vi "numberOptions.vi"(8 "Error In":errorcluster, 11 "QLocale In":refnum<class "QLocale.lvclass">) -> (0 "Error Out":errorcluster, 2 "Value":T1 items=["DefaultNumberOptions"=0, "OmitGroupSeparator"=1, "RejectGroupSeparator"=2, "OmitLeadingZeroInExponent"=4, "RejectLeadingZeroInExponent"=8, "IncludeTrailingZeroesAfterDot"=16, "RejectTrailingZeroesAfterDot"=32], 3 "QLocale Out":refnum<class "QLocale.lvclass">)   [LabVIEW 2014, in "QLocale.lvclass"]
doc: "LabVIEW-specific documentation is not yet available. See <b>https://doc.qt.io/qt-5/qlocale.html#numberOptions</b>"
uses:
  QLocale.lvclass
  NumberOption.ctl
  LQSerialData/LQSerialData.lvclass/LQSerialData.ctl
  LQ Core.lvlib
  LQSerialData/LQSerialData.lvclass
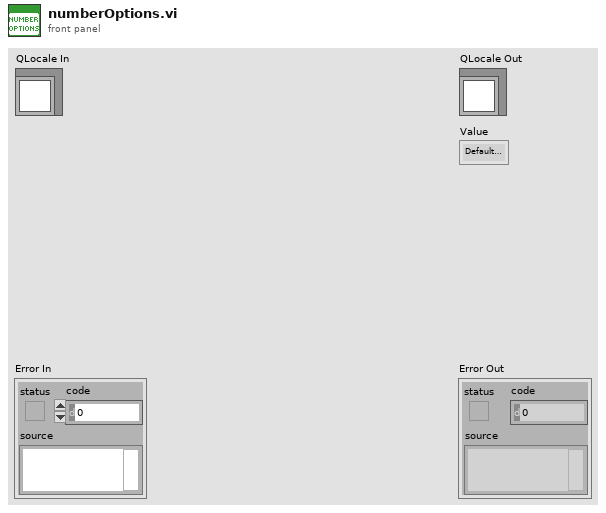
[diagram p1: front panel]
types:
  T1 = typedef "QLocale.lvclass/NumberOption.ctl" = i32
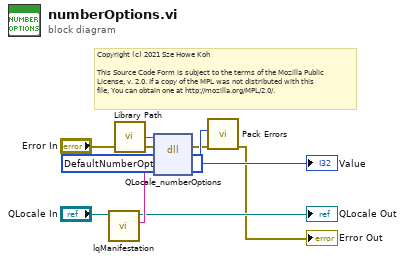
[diagram p0: block diagram]
diagram:
  w8 = T1 0 items=["DefaultNumberOptions"=0, "OmitGroupSeparator"=1, "RejectGroupSeparator"=2, "OmitLeadingZeroInExponent"=4, "RejectLeadingZeroInExponent"=8, "IncludeTrailingZeroesAfterDot"=16, "RejectTrailingZeroesAfterDot"=32] ("retVal")
  # "Copyright (c) 2021 Sze Howe Koh\n\nThis Source Code Form is subject to the terms of the Mozilla Public\nLicense, v. 2.0. If a copy of the MPL was not distributed with this\nfile, You can obtain one at http://mozilla.org/MPL/2.0/."
  n1 = call "lqManifestation.vi"("LQSerialData in"="QLocale In") -> ("Manifestation"=w7:string, "LQSerialData out"=→"QLocale Out":refnum<class "QLocale.lvclass">)  [unwired: 9 in]
  n2 = call "Library Path.vi"() -> ("Library Path"=w4:path)
  n3 = dll-call lib="?" fn="QLocale_numberOptions"(path in=w4, error in="Error In", "_retVal"=w8, "_instance"=w7) -> (error out=w2:errorcluster, w3:i32, "_retVal"=→"Value":i32)  [unwired: 2 in, 1 out]
  n4 = call "Pack Errors.vi"("Error In"=w2, "Error Code"=w3) -> ("Error Out"=→"Error Out":errorcluster)  [unwired: 9 in]
